vi "Register to Discovery Service.vi"(0 "gRPC ID in":T2, 5 "port number":i32, 7 "measurement plugin service in":refnum<class "Measurement Plugin Service.lvclass">, 9 "measurement service in":refnum<class "IMeasurement Service.lvclass">[](array[class]), 11 "error in":errorcluster) -> (4 "gRPC ID out":T2, 6 "response data":T1, 8 "measurement plugin service out":refnum<class "Measurement Plugin Service.lvclass">, 10 "measurement service out":refnum<class "IMeasurement Service.lvclass">[](array[class]), 15 "error out":errorcluster)   [LabVIEW 2021, in "NI Measurement Plug-In SDK.lvlib"]
uses:
  NI Measurement Plug-In SDK.lvlib
  <vilib>/gRPC/LabVIEW gRPC Library/Shared/grpcId.ctl
  gRPC/Generated APIs/ni/measurementlink/discovery/v1/RPC Messages/ni_measurementlink_discovery_v1_RegisterServiceResponse.ctl
  Measurement Plugin Service/Measurement Plugin Service.lvclass
  IMeasurement Service/IMeasurement Service.lvclass
  gRPC/Generated APIs/ni/measurementlink/discovery/v1/RPC Messages/ni_measurementlink_discovery_v1_RegisterServiceRequest.ctl
  gRPC/Generated APIs/ni/measurementlink/discovery/v1/RPC Messages/ni_measurementlink_discovery_v1_ServiceDescriptor.ctl
  gRPC/Generated APIs/ni/measurementlink/discovery/v1/RPC Messages/ni_measurementlink_discovery_v1_ServiceDescriptor_AnnotationsEntry.ctl
  gRPC/Generated APIs/ni/measurementlink/discovery/v1/RPC Messages/ni_measurementlink_discovery_v1_ServiceLocation.ctl
  gRPC/Generated APIs/ni/measurementlink/discovery/v1/ni.measurementlink.discovery.v1.api.lvlib
  <vilib>/gRPC/LabVIEW gRPC Library/grpc-lvsupport-release.lvlib
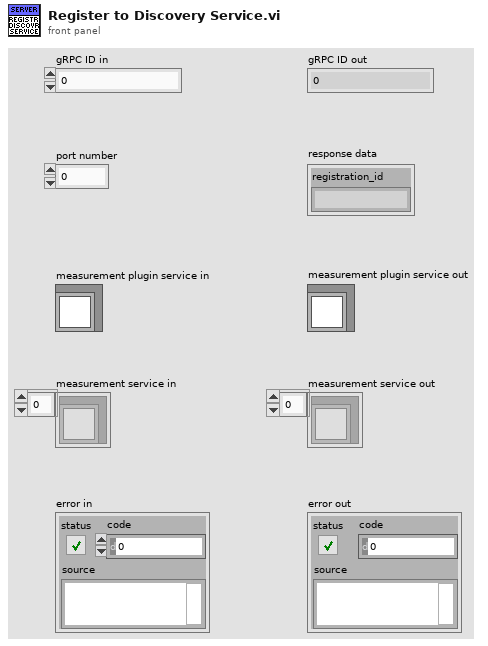
[diagram p1: front panel]
types:
  T1 = typedef "ni.measurementlink.discovery.v1.api.lvlib/ni_measurementlink_discovery_v1_RegisterServiceResponse.ctl" = cluster{"registration_id":string}
  T2 = typedef "grpc-lvsupport-release.lvlib/grpcId.ctl" = u64
  T3 = typedef "ni.measurementlink.discovery.v1.api.lvlib/ni_measurementlink_discovery_v1_RegisterServiceRequest.ctl" = cluster{"service_description":T4, "location":T6}
  T4 = typedef "ni.measurementlink.discovery.v1.api.lvlib/ni_measurementlink_discovery_v1_ServiceDescriptor.ctl" = cluster{"display_name":string, "description_url":string, "provided_interfaces":string[], "service_class":string, "annotations":T5[], "versions":string[]}
  T5 = typedef "ni.measurementlink.discovery.v1.api.lvlib/ni_measurementlink_discovery_v1_ServiceDescriptor_AnnotationsEntry.ctl" = cluster{"key":string, "value":string}
  T6 = typedef "ni.measurementlink.discovery.v1.api.lvlib/ni_measurementlink_discovery_v1_ServiceLocation.ctl" = cluster{"location":string, "insecure_port":string, "ssl_authenticated_port":string}
  T7 = typedef "NI Measurement Plug-In SDK.lvlib/Service Descriptor.ctl" = cluster{"measurement details":T8, "description URL":string, "service class":string, "measurement annotations":T9[]}
  T8 = typedef "NI Measurement Plug-In SDK.lvlib/Measurement Details.ctl" = cluster{"display name":string, "version":string}
  T9 = typedef "NI Measurement Plug-In SDK.lvlib/Measurement Annotation.ctl" = cluster{"key":string, "value":string}
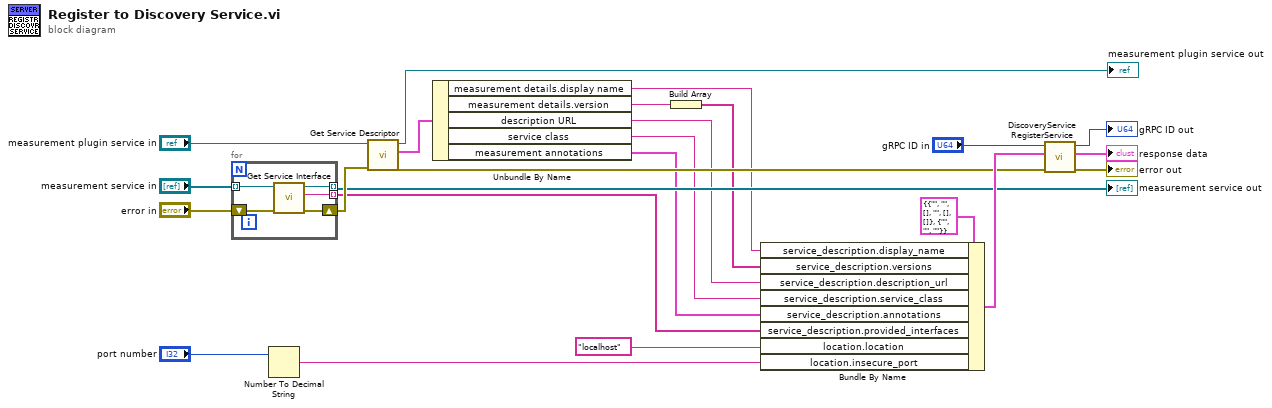
[diagram p0: block diagram]
diagram:
  n1 = for {
    tunnel: "measurement service in" -> [w29] mode=indexing
    tunnel: [w28] -> w5 mode=indexing
    shift-right: [w26] -> w12
    shift-left: "error in" -> [w27]
    tunnel: [w25] -> w10 mode=indexing
    n2 = call-dynamic "Get Service Interface.vi"("error in"=w27, "measurement service in"=w29) -> ("error out"=w26:errorcluster, "service interface"=w28:string, "measurement service out"=w25:refnum<class "IMeasurement Service.lvclass">)  [unwired: 7 in]
  }
  "measurement service out" <- w10
  n3 = Number To Decimal String(number="port number") -> (decimal integer string=w24:string)  [unwired: 1 in]
  n4 = call "Get Service Descriptor.vi"("error in"=w12, "measurement plugin service in"="measurement plugin service in") -> ("error out"=w14:errorcluster, "service descriptor"=w9:T7, "measurement plugin service out"=→"measurement plugin service out":refnum<class "Measurement Plugin Service.lvclass">)  [unwired: 7 in]
  n5 = Unbundle By Name(w9) -> ("measurement details.display name"=w3:string, "measurement details.version"=w2:string, "description URL"=w8:string, "service class"=w7:string, "measurement annotations"=w4:T9[])
  n6 = Build Array(w2) -> (w1:string[])
  n7 = Bundle By Name(cluster=T3 {"service_description"={"display_name"="", "description_url"="", "provided_interfaces"=[], "service_class"="", "annotations"=[], "versions"=[]}, "location"={"location"="", "insecure_port"="", "ssl_authenticated_port"=""}} ("Request Data"), "service_description.display_name"=w3, "service_description.versions"=w1, "service_description.description_url"=w8, "service_description.service_class"=w7, "service_description.annotations"=w4, "service_description.provided_interfaces"=w5, "location.location"="localhost", "location.insecure_port"=w24) -> (w20:T3)
  n8 = call "DiscoveryService RegisterService.vi"("error in"=w14, "Request Data"=w20, "gRPC ID"="gRPC ID in") -> ("error out"=→"error out":errorcluster, "Response Data"=→"response data":T1, "gRPC ID out"=→"gRPC ID out":T2)  [unwired: 6 in]
